vi "InvalidTag_ReturnsError.vi"() -> (0 "error out":errorcluster)   [LabVIEW 2019, in "ResultTreeTest.lvlib" / "SetIcon.lvlib"]
uses:
  SetIcon.lvlib
  ResultTree/Icon.ctl
  ResultTree/ResultTree.lvclass
  Assertion/Assertion.lvlib
panel:
  in  "Tree":string(tree)
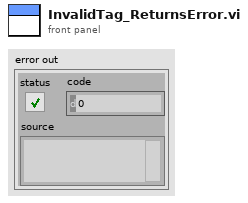
[diagram p1: front panel]
types:
  T1 = typedef "ResultTree.lvclass/Icon.ctl" = enum16{"None", "Passed", "Failed", "Error"}
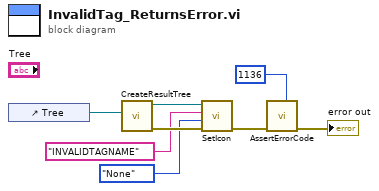
[diagram p0: block diagram]
diagram:
  n1 = control-ref of="Tree"() -> (w6:refnum<vi>)
  n2 = call "CreateResultTree.vi"("Tree Refnum"=w6) -> ("error out"=w8:errorcluster, "ResultTree out"=w7:refnum<class "ResultTree.lvclass">)  [unwired: 9 in]
  n3 = call "SetIcon.vi"("error in (no error)"=w8, "Icon"=Icon."None", "Tag Name"="INVALIDTAGNAME", "ResultTree in"=w7) -> ("error out"=w3:errorcluster)  [unwired: 6 in, 1 out]
  n4 = call "AssertErrorCode.vi"("Expected"=1136, "error in (no error)"=w3) -> ("error out"=→"error out":errorcluster)  [unwired: 9 in]
